vi "circlefilter.vi"(11 "Circle Diameter":dbl) -> (2 "Filter Weights":sgl[][](array[numeric]), 3 "Image border size":dbl)   [LabVIEW 2019]
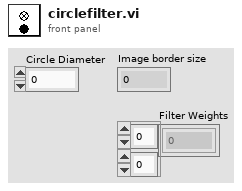
[diagram p1: front panel]
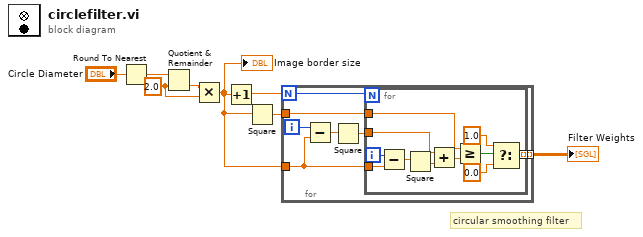
[diagram p0: block diagram]
diagram:
  w3 = 2.0 ("y")
  # "circular smoothing filter"
  n1 = Round To Nearest(number="Circle Diameter") -> ()  [unwired: 1 out]
  n2 = Quotient & Remainder(x="Circle Diameter", y=w3) -> (floor(x/y)=w4:dbl)  [unwired: 1 out]
  n3 = Multiply(x=w4, y=w3) -> (x*y=w1:dbl)
  "Image border size" <- w1
  n4 = Increment(x=w1) -> (x+1=w2:dbl)
  n5 = Square(x=w1) -> (x^2=w7:dbl)
  n6 = for {
    N: w2 -> [w10]
    tunnel: w1 -> [w13]
    tunnel: [w9] -> w6 mode=indexing
    tunnel: w7 -> [w8]
    i -> [w14]
    n7 = Subtract(x=w14, y=w13) -> (x-y=w12:dbl)
    n8 = Square(x=w12) -> (x^2=w11:dbl)
    n9 = for {
      N: w10 -> [_]
      tunnel: w13 -> [w25]
      tunnel: w11 -> [w21]
      tunnel: [w16] -> w9 mode=indexing
      tunnel: w8 -> [w15]
      i -> [w24]
      n10 = Subtract(x=w24, y=w25) -> (x-y=w23:dbl)
      n11 = Square(x=w23) -> (x^2=w22:dbl)
      n12 = Add(x=w21, y=w22) -> (x+y=w20:dbl)
      n13 = Greater Or Equal?(x=w15, y=w20) -> (x >= y?=w19:bool)
      n14 = Select(t=sgl 1.0, s=w19, f=sgl 0.0) -> (s? t:f=w16:sgl)
    }
  }
  "Filter Weights" <- w6
